vi "Global_Constant.vi"() -> ()   [LabVIEW 2020]
panel:
  in  "ADJ CUST":string[][](table)=[["1"], [""]]
  in  "Use ADJ":string[][](table)=[["10210-1"], ["10210-2"], ["10223-0"], ["10234-0"], ["10236-0"], ["10511-3"], ["20109-0"], ["20202-0"], ["20203-0"], ["20204-0"], ["20302-0"], ["20303-0"], ["20406-0"], ["20408-0"], ["20409-0"], ["20411-1"], ["20411-4"], ["20412-1"], ["20412-2"], ["20413-0"], ["20414-0"]]
  out "Display Sys":string[][](table)=[["Check", "Check", "Check", "Check", "단능형", "Check", "Analog", "Digital", "Digital"], ["Digital", "Digital", "Digital", "Digital", "지시형", "Digital", "", "", "Analog"], ["Analog(1/1)", "Dial", "Dial", "Dial", "프리셋형", "Analog", "", "", ""], ["Analog(1/2)", "Vernier", "", "Analog", "", "", "", "", ""], ["Analog(1/5)", "", "", "Vernier", "", "", "", "", ""], ["Analog(1/10)", "", "", "", "", "", "", "", ""]]
  out "Unit Set":string[][](table)=[["nm", "μg", "mN", "mN·m", "Pa", "atm", "nHz", "as", "nA", "nV", "nΩ", "abH", "aF", "mW", "㎟", "℃", "˚", "실수", "r/min", "ppm/℃"], ["μm", "mg", "cN", "cN·m", "hPa", "Pa abs.", "μHz", "fs", "μA", "μV", "μΩ", "μH", "fF", "W", "㎠", "℉", "´", "%", "% R.H.", "%/℃"], ["mm", "g", "N", "N·m", "kPa", "hPa abs.", "mHz", "ps", "mA", "mV", "mΩ", "mH", "pF", "kW", "㎡", "K", "˝", "ppm", "lux", "/℃"], ["cm", "kg", "kN", "kgf·m", "MPa", "kPa abs.", "Hz", "ns", "A", "V", "Ω", "H", "nF", "", "", "", "rad", "Div.", "dB", ""], ["m", "ton", "lbf", "gf·cm", "mbar", "MPa abs.", "kHz", "μs", "", "kV", "kΩ", "", "μF", "", "", "", "mm/m", "", "dB re 1 V/Pa", ""], ["inch", "oz", "gf", "kgf·cm", "bar", "mbar abs.", "MHz", "ms", "", "", "MΩ", "", "mF", "", "", "", "μm/m", "", "dBm", ""], ["feet", "lb", "kgf", "ozf·in", "mmHg", "bar abs.", "GHz", "s", "", "", "GΩ", "", "F", "", "", "", "cm/m", "", "P.F", ""], ["in", "", "ton.f", "lbf·in", "cmHg", "psi abs.", "THz", "min", "", "", "TΩ", "", "", "", "", "", "", "", "×", ""], ["ft", "", "ozf", "lbf·ft", "psi", "kgf/㎠ abs.", "", "h", "", "", "", "", "", "", "", "", "", "", "", ""], ["", "", "", "", "inH2O", "", "", "", "", "", "", "", "", "", "", "", "", "", "", ""], ["", "", "", "", "mmH2O", "", "", "", "", "", "", "", "", "", "", "", "", "", "", ""], ["", "", "", "", "cmH2O", "", "", "", "", "", "", "", "", "", "", "", "", "", "", ""], ["", "", "", "", "kgf/㎠", "", "", "", "", "", "", "", "", "", "", "", "", "", "", ""], ["", "", "", "", "kgf/㎡", "", "", "", "", "", "", "", "", "", "", "", "", "", "", ""], ["", "", "", "", "inHg", "", "", "", "", "", "", "", "", "", "", "", "", "", "", ""], ["", "", "", "", "atm", "", "", "", "", "", "", "", "", "", "", "", "", "", "", ""], ["", "", "", "", "N/㎠", "", "", "", "", "", "", "", "", "", "", "", "", "", "", ""], ["", "", "", "", "", "", "", "", "", "", "", "", "", "", "", "", "", "", "", ""], ["", "", "", "", "", "", "", "", "", "", "", "", "", "", "", "", "", "", "", ""], ["", "", "", "", "", "", "", "", "", "", "", "", "", "", "", "", "", "", "", ""], ["", "", "", "", "", "", "", "", "", "", "", "", "", "", "", "", "", "", "", ""], ["", "", "", "", "", "", "", "", "", "", "", "", "", "", "", "", "", "", "", ""], ["", "", "", "", "", "", "", "", "", "", "", "", "", "", "", "", "", "", "", ""], ["", "", "", "", "", "", "", "", "", "", "", "", "", "", "", "", "", "", "", ""]]
  in  "MK Proc":string[][](table)=[["10206-0", "Type_0"], ["10209-0", "Type_0"], ["10210-1", "Type_3"], ["10210-2", "Type_3"], ["10211-0", "Type_3"], ["10214-0", "Type_0"], ["10216-0", "Type_0"], ["10223-0", "Type_3"], ["10227-0", "Type_0"], ["10228-2", "Type_3"], ["10229-0", "Type_3"], ["10232-1", "Type_0"], ["10232-2", "Type_0"], ["10233-0", "Type_0"], ["10234-0", "Type_0"], ["10235-1", "Type_3"], ["10235-2", "Type_3"], ["10236-0", "Type_0"], ["10304-2", "Type_0"], ["10311-1", "Type_0"], ["10311-2", "Type_0"], ["10404-0", "Type_0"], ["10405-0", "Type_0"], ["10407-0", "Type_0"], ["10413-0", "Type_0"], ["10503-0", "Type_0"], ["10504-1", "Type_0"], ["10511-1", "Type_0"], ["10511-2", "Type_0"], ["10511-3", "Type_3"], ["10512-0", "Type_3"], ["10517-0", "Type_0"], ["10601-1", "Type_0"], ["10601-3", "Type_0"], ["10603-1", "Type_0"], ["10603-2", "Type_0"], ["10604-1", "Type_0"], ["10604-2", "Type_3"], ["10605-1", "Type_0"], ["10605-2", "Type_0"], ["10609-1", "Type_0"], ["10609-2", "Type_0"], ["10610-0", "Type_0"], ["10611-0", "Type_0"], ["10612-1", "Type_3"], ["10612-2", "Type_3"], ["10613-1", "Type_0"], ["20109-0", "Type_0"], ["20116-1", "Type_0"], ["20116-2", "Type_0"], ["20202-0", "Type_0"], ["20204-0", "Type_0"], ["20302-0", "Type_0"], ["20303-0", "Type_0"], ["20406-0", "Type_0"], ["20408-0", "Type_0"], ["20409-0", "Type_0"], ["20411-1", "Type_0"], ["20411-4", "Type_0"], ["20412-1", "Type_0"], ["20412-2", "Type_0"], ["20413-0", "Type_0"], ["20414-0", "Type_0"], ["40419-0", "Type_1"]]
  # "Type_0 : 일반\nType_1 : 다기능(전기 등)\nType_3 : 최대범위, 최소범위"
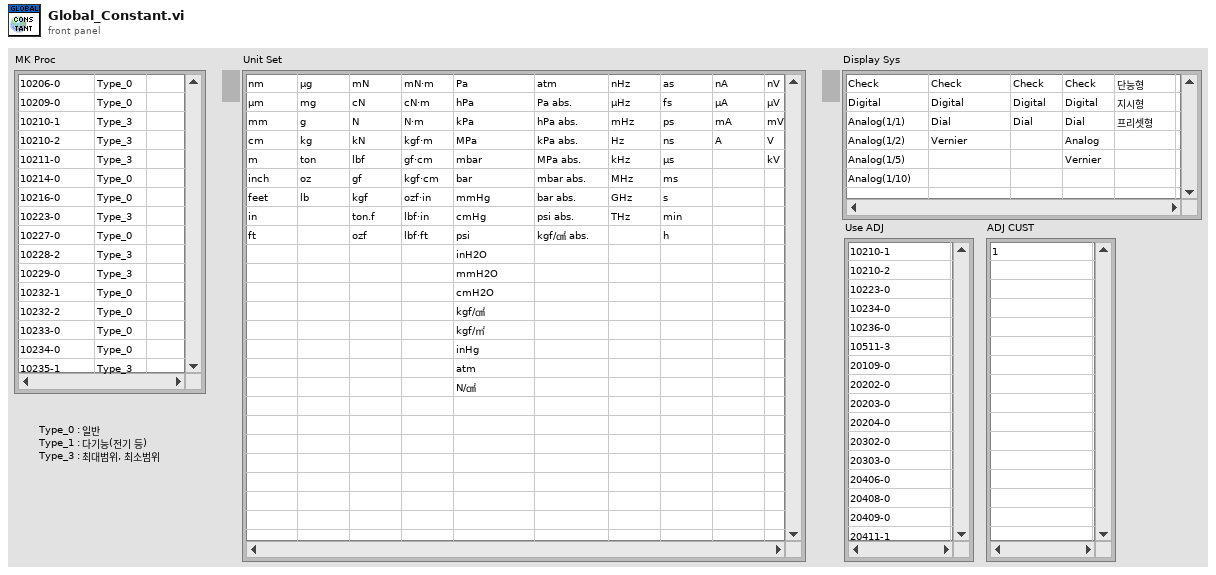
[diagram p1: front panel]
diagram:
